vi "Labview_OPC_UA_Server.vi"() -> ()   [LabVIEW 2025]
uses:
  <vilib>/OPCUA/controls/NodeId.ctl
  <vilib>/OPCUA/controls/Data Type.ctl
  <vilib>/OPCUA/server/Create2.vi
  <vilib>/OPCUA/NI OPC UA Server.lvlib
panel:
  out "item node ID 2":T1
  out "item node ID":T1
  out "Item node ID":string
  out "Server endpoint url":string
  in  "Stop":bool
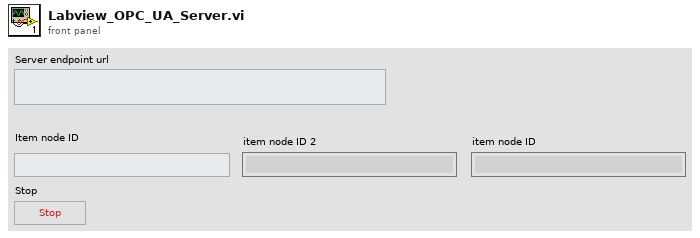
[diagram p1: front panel]
types:
  T1 = typedef "NodeId.ctl" = string
  T2 = typedef "Data Type.ctl" = u16
  T3 = cluster{"name":string, "data type":T2, "access level":u16, "description":string}
  T4 = typedef "OPC UA Server Refnum.ctl" = refnum<k21>
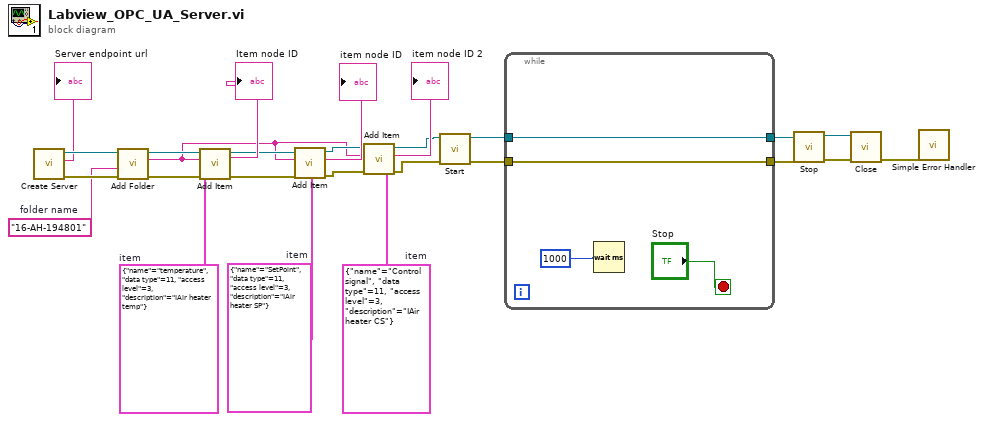
[diagram p0: block diagram]
diagram:
  w2 = T3 {"name"="Control signal", "data type"=11, "access level"=3, "description"="IAir heater CS"}  # item
  w3 = T3 {"name"="SetPoint", "data type"=11, "access level"=3, "description"="IAir heater SP"}  # item
  w19 = T3 {"name"="temperature", "data type"=11, "access level"=3, "description"="IAir heater temp"}  # item
  w20 = "16-AH-194801"  # folder name
  n1 = call-poly <vilib>:"Create Server.vi"() -> ("error out"=w26:errorcluster, "server endpoint URL"=→"Server endpoint url":string, "OPC UA server refnum out"=w17:T4)  [unwired: 9 in]
  n2 = call <vilib>:"Add Folder.vi"("error in (no error)"=w26, "folder name"=w20, "OPC UA server refnum in"=w17) -> ("error out"=w25:errorcluster, "folder node ID"=w1:T1, "OPC UA server refnum out"=w16:T4)  [unwired: 5 in]
  n3 = call <vilib>:"Add Item.vi"("error in (no error)"=w25, "item"=w19, "parent folder node ID"=w1, "OPC UA server refnum in"=w16) -> ("error out"=w11:errorcluster, "item node ID"=→"Item node ID":T1, "OPC UA server refnum out"=w6:T4)  [unwired: 3 in, 1 out]
  n4 = call <vilib>:"Add Item.vi"("error in (no error)"=w11, "item"=w3, "parent folder node ID"=w1, "OPC UA server refnum in"=w6) -> ("error out"=w10:errorcluster, "item node ID"=→"item node ID":T1, "OPC UA server refnum out"=w5:T4)  [unwired: 3 in, 1 out]
  n5 = call <vilib>:"Add Item.vi"("error in (no error)"=w10, "item"=w2, "parent folder node ID"=w1, "OPC UA server refnum in"=w5) -> ("error out"=w9:errorcluster, "item node ID"=→"item node ID 2":T1, "OPC UA server refnum out"=w4:T4)  [unwired: 3 in, 1 out]
  n6 = call <vilib>:"Start.vi"("error in (no error)"=w9, "OPC UA server refnum in"=w4) -> ("error out"=w24:errorcluster, "OPC UA server refnum out"=w15:T4)  [unwired: 7 in, 1 out]
  n7 = while {
    tunnel: w24 -> [w28]
    tunnel: [w28] -> w23
    tunnel: w15 -> [w27]
    tunnel: [w27] -> w14
    stop <- "Stop" stop-if-true
    n8 = Wait (ms)(milliseconds to wait=u32 1000) -> ()  [unwired: 1 out]
  }
  n9 = call <vilib>:"Stop.vi"("error in (no error)"=w23, "OPC UA server refnum in"=w14) -> ("error out"=w22:errorcluster, "OPC UA server refnum out"=w13:T4)  [unwired: 8 in]
  n10 = call <vilib>:"Close.vi"("error in (no error)"=w22, "OPC UA server refnum in"=w13) -> ("error out"=w21:errorcluster)  [unwired: 9 in]
  n11 = call <vilib>:"Simple Error Handler.vi"("error in (no error)"=w21) -> ()  [unwired: 4 in, 5 out]
